vi "Byte Buffer.Set Byte Order.vi"(8 "error in (no error)":errorcluster, 10 "byte order":T1(ring), 11 "Byte Buffer in":refnum<class "Byte Buffer.lvclass">) -> (0 "error out":errorcluster, 3 "Byte Buffer out":refnum<class "Byte Buffer.lvclass">)   [LabVIEW 2016, in "VeriStand Data.lvlib" / "Byte Buffer.lvclass"]
doc: "Gets the raw string buffer from the provided Byte Buffer class."
uses:
  Byte Buffer.lvclass
  Byte Buffer.lvclass/Byte Buffer.ctl
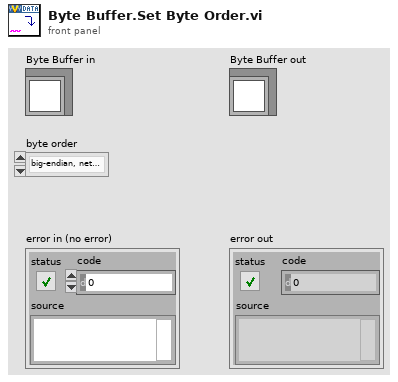
[diagram p1: front panel]
types:
  T1 = enum16{"big-endian, network order", "native, host order", "little-endian"}
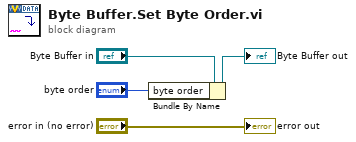
[diagram p0: block diagram]
diagram:
  n1 = Bundle By Name(cluster="Byte Buffer in", "byte order"="byte order") -> (→"Byte Buffer out":refnum<class "Byte Buffer.lvclass">)
  "error out" <- "error in (no error)"
